vi "Meas Result Fill Phase Selector.vi"(1 "results data":T1, 2 "res pid":refnum<vi>) -> (0 "phase index (default: 0)":u16)   [LabVIEW 2013]
doc: "Fills list of phase selector based on phase count available in result data."
uses:
  Meas Results.ctl
  bridge/Bridge Frequency Readings Data.ctl
  drivers/TWM client/Meas Proc QWTB Spectrum Data.ctl
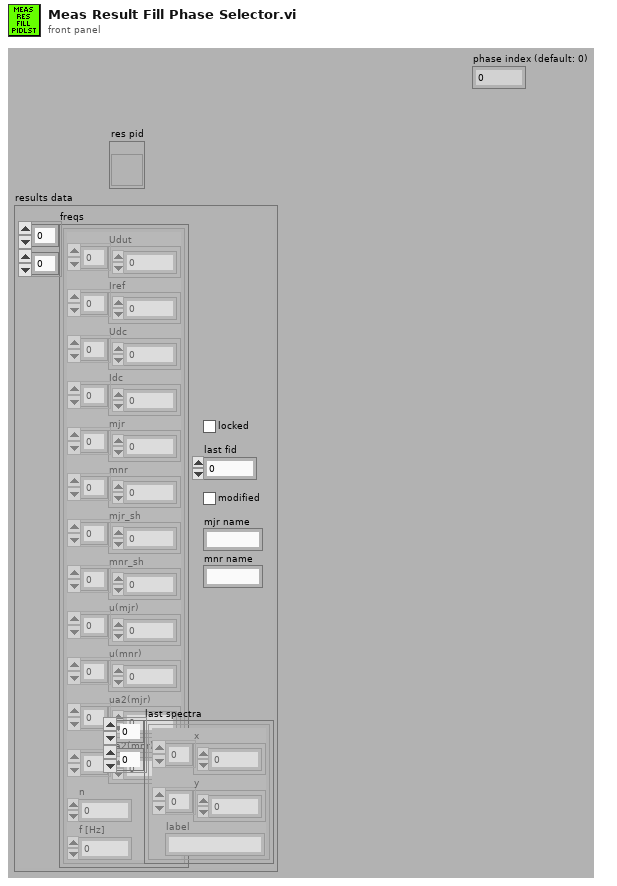
[diagram p1: front panel]
types:
  T1 = typedef "Meas Results.ctl" = cluster{"freqs":T2[][], "locked":bool, "last fid":i32, "modified":bool, "mjr name":string, "mnr name":string, "last spectra":T3[][]}
  T2 = typedef "Bridge Frequency Readings Data.ctl" = cluster{"Udut":dbl[], "Iref":dbl[], "Udc":dbl[], "Idc":dbl[], "mjr":dbl[], "mnr":dbl[], "mjr_sh":dbl[], "mnr_sh":dbl[], "u(mjr)":dbl[], "u(mnr)":dbl[], "ua2(mjr)":dbl[], "ua2(mnr)":dbl[], "n":i32, "f [Hz]":dbl}
  T3 = typedef "Meas Proc QWTB Spectrum Data.ctl" = cluster{"x":sgl[], "y":sgl[], "label":string}
  T4 = enum8{"Enabled", "Disabled", "Disabled and Grayed Out"}
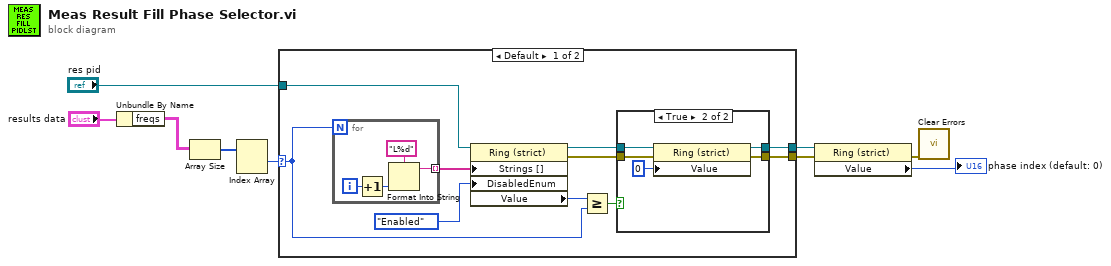
[diagram p0: block diagram]
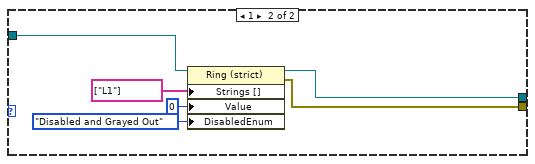
[diagram p3: hidden frame]
diagram:
  n1 = Unbundle By Name("results data") -> ("freqs"=w8:T2[][])
  n2 = Array Size(array=w8) -> (size(s)=w7:i32[])
  n3 = Index Array(array=w7) -> (element #1=w6:i32)  [unwired: 2 in, 1 out]
  n4 = case shown="Default" w6 {
    selector: w6 -> [w15 _]
    tunnel: "res pid" -> [w18 w36]
    tunnel: [w11 w31] -> w4
    tunnel: [w10 w32] -> w3
    frame Default {
      n5 = for {
        N: w15 -> [_]
        tunnel: [w27] -> w19 mode=indexing
        i -> [w30]
        n6 = Increment(x=w30) -> (x+1=w29:i32)
        n7 = Format Into String(format string="L%d", w29) -> (resulting string=w27:string)  [unwired: 2 in, 1 out]
      }
      n8 = property class="Ring (strict)"(reference=w18, "Strings []"=w19, "DisabledEnum"=T4."Enabled" ("Disabled")) -> (reference out=w12:refnum<vi>, error out=w13:errorcluster, "Value"=w16:u16)  [unwired: 1 in]
      n9 = Greater Or Equal?(x=w16, y=w15) -> (x >= y?=w14:bool)
      n10 = case shown="True" w14 {
        tunnel: w13 -> [w21 w26]
        tunnel: w12 -> [w20 w25]
        tunnel: [w21 w23] -> w11
        tunnel: [w20 w22] -> w10
        frame False {
        }
        frame True {
          n11 = property class="Ring (strict)"(reference=w25, error in=w26, "Value"=u16 0) -> (reference out=w22:refnum<vi>, error out=w23:errorcluster)
        }
      }
    }
    frame 1 {
      n12 = property class="Ring (strict)"(reference=w36, "Strings []"=string[] ["L1"], "Value"=u16 0, "DisabledEnum"=T4."Disabled and Grayed Out" ("Disabled")) -> (reference out=w32:refnum<vi>, error out=w31:errorcluster)  [unwired: 1 in]
    }
  }
  n13 = property class="Ring (strict)"(reference=w3, error in=w4) -> (error out=w2:errorcluster, "Value"=→"phase index (default: 0)":u16)  [unwired: 1 out]
  n14 = call <vilib>:"Clear Errors.vi"("error in (no error)"=w2) -> ()  [unwired: 6 in, 1 out]
